vi "DT_Triangle Manager_Check Ghost_Core.vi"(11 "Triangle":i32[](array[numeric])) -> (2 "ghost tri?":bool)   [LabVIEW 2017, in "NI_AAL_Geometry.lvlib"]
uses:
  <vilib>/Analysis/NI_AAL_Geometry.lvlib
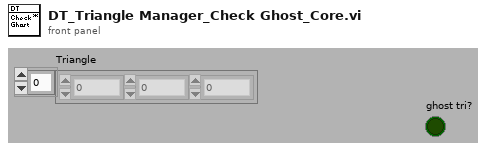
[diagram p1: front panel]
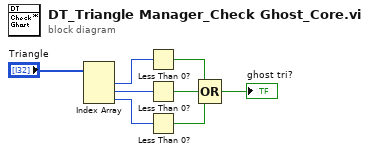
[diagram p0: block diagram]
diagram:
  n1 = Index Array(array="Triangle") -> (element #1=w7:i32, element #2=w6:i32, element #3=w5:i32)  [unwired: 3 in]
  n2 = Less Than 0?(x=w7) -> (x < 0?=w4:bool)
  n3 = Less Than 0?(x=w6) -> (x < 0?=w3:bool)
  n4 = Less Than 0?(x=w5) -> (x < 0?=w2:bool)
  n5 = Compound Arithmetic op=OR(w4, w3, w2) -> (→"ghost tri?":bool)
